vi "GetMDPtrQueue.vi"(8 "error in (no error)":errorcluster, 10 "CacheSize":i32, 11 "MDPtrMgr in":refnum<class "MDPtrMgr.lvclass">) -> (0 "error out":errorcluster, 1 "Total MDPtrQueue":T1, 2 "MDPtrQueue":T1, 3 "MDPtrMgr out":refnum<class "MDPtrMgr.lvclass">)   [LabVIEW 2017, in "MDPtr.lvlib" / "MDPtrMgr.lvclass"]
uses:
  MDPtrMgr.lvclass
  MDPtr TypeDef/MDPtr Queue.ctl
  MDPtr TypeDef/MDPtr DataFrame-Memory.ctl
  MDPtr TypeDef/MDPtr DataFrame-Common.ctl
  <vilib>/Utility/Data Type/Type Definitions/Data Type.ctl
  MDPtrMgr.lvclass/MDPtrMgr.ctl
  MDPtr.lvlib
  <vilib>/Utility/Data Type/NI_Data Type.lvlib
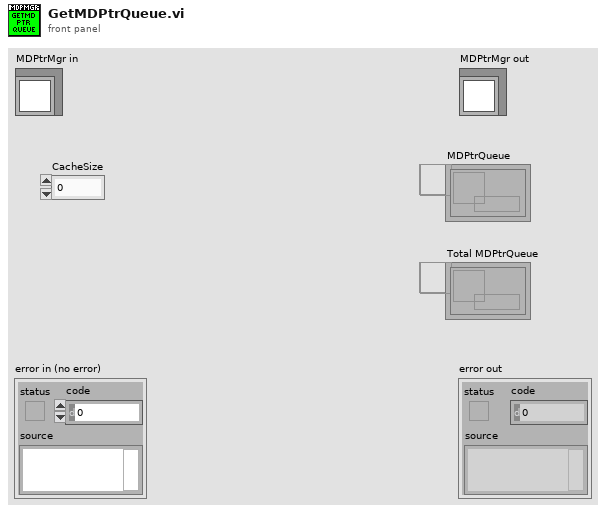
[diagram p1: front panel]
types:
  T1 = typedef "MDPtr.lvlib/MDPtr Queue.ctl" = refnum<queue>
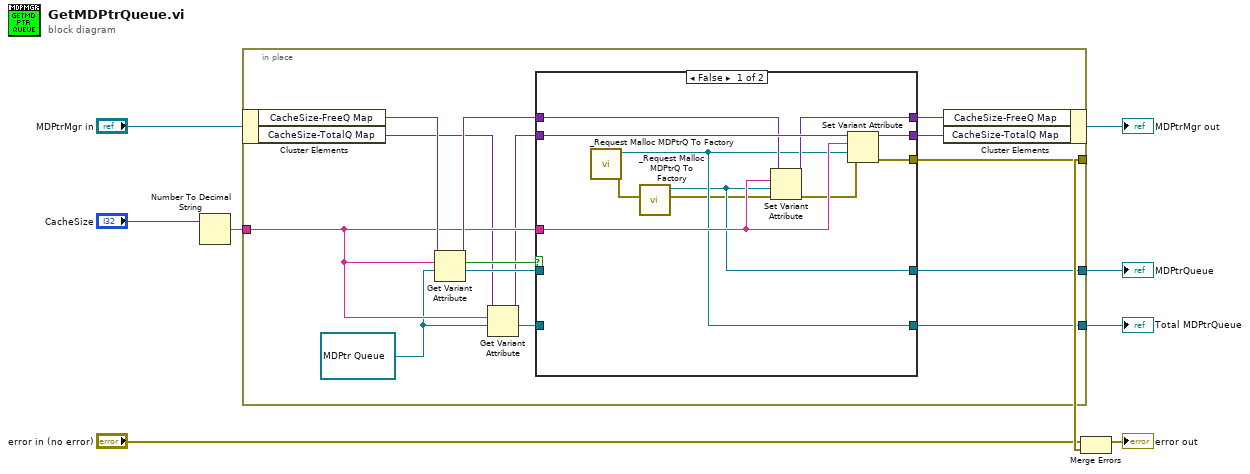
[diagram p0: block diagram]
diagram:
  n1 = Number To Decimal String(number="CacheSize") -> (decimal integer string=w7:string)  [unwired: 1 in]
  n2 = in-place "In Place Element Structure" {
    in-place-border: w7 -> [w15]
    in-place-border: [w17] -> w6
    in-place-border: [w16] -> w5
    in-place-border: [w10] -> w3
    w14 = T1 refnum ("MDPtrQueue")
    n3 = in-place-cluster #1("MDPtrMgr in") -> ("CacheSize-FreeQ Map"=w23:variant, "CacheSize-TotalQ Map"=w13:variant)
    n4 = Get Variant Attribute(Variant=w23, name=w15, default value (empty Variant)=w14) -> (duplicate Variant=w21:variant, found=w19:bool, value=w18:T1)  [unwired: 1 in, 1 out]
    n5 = Get Variant Attribute(Variant=w13, name=w15, default value (empty Variant)=w14) -> (duplicate Variant=w12:variant, value=w11:T1)  [unwired: 1 in, 2 out]
    n6 = case shown="False" w19 {
      tunnel: [w34 w38] -> w22
      tunnel: w12 -> [w33 w38]
      tunnel: w21 -> [w32 w37]
      tunnel: [w31 w37] -> w20
      tunnel: w15 -> [w30 _]
      tunnel: w18 -> [_ w36]
      tunnel: [w28 w36] -> w17
      tunnel: [w29 w35] -> w16
      tunnel: w11 -> [_ w35]
      tunnel: [w24 _] -> w10
      frame False {
        n7 = call "_Request Malloc MDPtrQ To Factory.vi"() -> ("error out"=w27:errorcluster, "MDPtrQueue"=w29:T1)  [unwired: 10 in]
        n8 = call "_Request Malloc MDPtrQ To Factory.vi"("error in (no error)"=w27) -> ("error out"=w26:errorcluster, "MDPtrQueue"=w28:T1)  [unwired: 9 in]
        n9 = Set Variant Attribute(Variant=w32, name=w30, value=w28, error in=w26) -> (Variant out=w31:variant, error out=w25:errorcluster)  [unwired: 1 out]
        n10 = Set Variant Attribute(Variant=w33, name=w30, value=w29, error in=w25) -> (Variant out=w34:variant, error out=w24:errorcluster)  [unwired: 1 out]
      }
      frame True {
      }
    }
    n11 = in-place-cluster #1("CacheSize-FreeQ Map"=w20, "CacheSize-TotalQ Map"=w22) -> (→"MDPtrMgr out":refnum<class "MDPtrMgr.lvclass">)
  }
  "MDPtrQueue" <- w6
  "Total MDPtrQueue" <- w5
  n12 = Merge Errors("error in (no error)", w3) -> (→"error out":errorcluster)
